vi "Tell Self.vi"(4 "Priority":bool, 10 "Msg":refnum<class "Msg.lvclass">, 11 "Base Actor in":refnum<class "Base Actor.lvclass">) -> (0 "Error out":errorcluster)   [LabVIEW 2025, in "jettl.lvlib" / "Actor.lvlib" / "Base Actor.lvclass"]
uses:
  Base Actor.lvclass
  Base Actor.lvclass/Base Actor.ctl
  Relation.ctl
  Actor.lvlib
  Error/Error.lvlib
  Teller/Teller.lvlib
  Msg/Msg.lvclass
  Attributes/Attributes/Attributes.lvclass
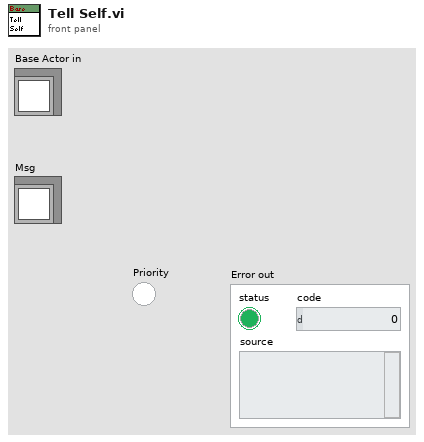
[diagram p1: front panel]
types:
  T1 = typedef "jettl.lvlib/Actor.lvlib/Msg Set.ctl" = set{refnum<class "Msg.lvclass">}
  T2 = typedef "jettl.lvlib/Actor.lvlib/Relation.ctl" = enum16{"Self", "Parent", "Child"}
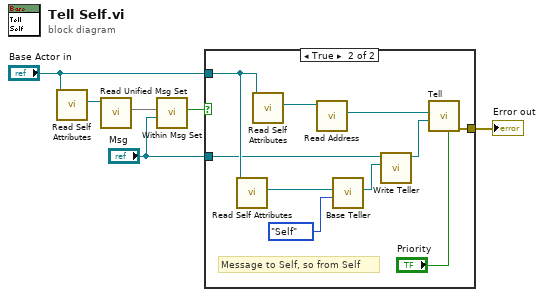
[diagram p0: block diagram]
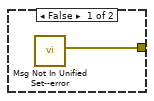
[diagram p2: hidden frame]
diagram:
  n1 = call-dynamic "Read Self Attributes.vi"("Base Actor in"="Base Actor in") -> ("Self Attributes"=w3:refnum<class "Attributes.lvclass">)  [unwired: 10 in]
  n2 = call-dynamic "Read Unified Msg Set.vi"("Attributes in"=w3) -> ("Unified Msg Set"=w2:T1)  [unwired: 10 in]
  n3 = call "Within Msg Set.vi"("Msg"="Msg", "Msg Set"=w2) -> ("Within Msg Set"=w6:bool)  [unwired: 9 in]
  n4 = case shown="True" w6 {
    tunnel: "Base Actor in" -> [_ w15]
    tunnel: "Msg" -> [_ w11]
    tunnel: [w7 w16] -> w1
    frame False {
      n5 = call "Msg Not In Unified Set--error.vi"() -> ("Error"=w7:errorcluster)  [unwired: 11 in]
    }
    frame True {
      # "Message to Self, so from Self"
      n6 = call-dynamic "Read Self Attributes.vi"("Base Actor in"=w15) -> ("Self Attributes"=w9:refnum<class "Attributes.lvclass">)  [unwired: 10 in]
      n7 = call-dynamic "Read Self Attributes.vi"("Base Actor in"=w15) -> ("Self Attributes"=w14:refnum<class "Attributes.lvclass">)  [unwired: 10 in]
      n8 = call-dynamic "Read Address.vi"("Attributes in"=w14) -> ("Address"=w13:refnum<user-event>)  [unwired: 10 in]
      n9 = call "Base Teller.vi"("Relation"=Relation."Self", "Self Attributes"=w9) -> ("Teller"=w12:refnum<class "Teller.lvclass">)  [unwired: 9 in]
      n10 = call-dynamic "Write Teller.vi"("Teller"=w12, "Msg in"=w11) -> ("Msg out"=w10:refnum<class "Msg.lvclass">)  [unwired: 9 in]
      n11 = call "Tell.vi"("Priority"="Priority", "Msg"=w10, "Address"=w13) -> ("Error out"=w16:errorcluster)  [unwired: 8 in]
    }
  }
  "Error out" <- w1
